vi "Write Error Pointer.vi"(8 "error in (no error)":errorcluster, 10 "error":errorcluster, 11 "Thread in":refnum<class "Thread.lvclass">) -> (0 "error out":errorcluster, 3 "Thread out":refnum<class "Thread.lvclass">)   [LabVIEW 2019, in "DSF Core.lvlib" / "Thread.lvclass"]
uses:
  Thread.lvclass
  Thread.lvclass/Thread.ctl
  Pointers/Error/Error Pointer.lvclass
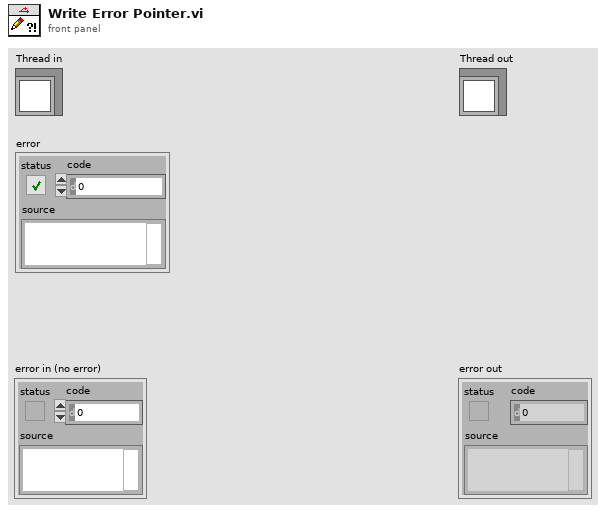
[diagram p1: front panel]
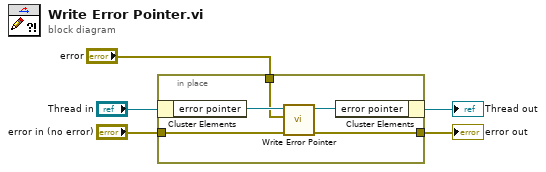
[diagram p0: block diagram]
diagram:
  n1 = in-place {
    in-place-border: [w7] -> w4
    in-place-border: "error in (no error)" -> [w10]
    in-place-border: "error" -> [w6]
    n2 = in-place-cluster #1("Thread in") -> ("error pointer"=w9:refnum<class "Error Pointer.lvclass">)
    n3 = call "Write Error Pointer.vi"("error in (no error)"=w10, "error"=w6, "Error Pointer in"=w9) -> ("error out"=w7:errorcluster, "Error Pointer in"=w8:refnum<class "Error Pointer.lvclass">)  [unwired: 7 in]
    n4 = in-place-cluster #1("error pointer"=w8) -> (→"Thread out":refnum<class "Thread.lvclass">)
  }
  "error out" <- w4
